vi "FPGA upload data to LEDs.vi"() -> ()   [LabVIEW 2016]
uses:
  Program Files (x86)/National Instruments/LabVIEW 2016/examples/roboRIO/Customized FPGA/Sub VIs/Utilities/Start Boolean.ctl
  <vilib>/Platform/TimedLoop/XDataNode/timing_clust.ctl
  <vilib>/Platform/TimedLoop/XDataNode/nitl_modes.ctl
  <vilib>/Platform/TimedLoop/XDataNode/wakeup.ctl
  <vilib>/rvi/Emulation/niFpgaGetClockAttributes.vi
  <vilib>/rvi/Emulation/niFpgaSctlEmulationGetInTimedLoop.vi
  <vilib>/rvi/Emulation/niFpgaEmulationReportErrorSimple.vi
  <vilib>/rvi/eio/common/nirviEmuTemplateMethod_errors.vi
  <vilib>/rvi/Emulation/niFpgaCriticalErrorInLSC.vi
  <vilib>/rvi/Emulation/niFpgaProcessEmulError.vi
  <vilib>/rvi/Emulation/niFpgaEmulationIsFPGAContextNoSignature.vi
  <vilib>/rvi/errors/niFpgaSetErrorForExecOnDevCompSimple.vi
  <vilib>/rvi/eio/common/nirviEmuReportErrorAndStop.vi
  <vilib>/rvi/DataTransferAndStorage/Container/Common/niFpgaContainerGetUniqueNameForEmu.vi
  <vilib>/rvi/FIFO/Fifo_Resource/nirvififoEmulationSetSize.vi
  <vilib>/rvi/FIFO/Fifo_Resource/nirviFifoEmulationQueueMgr.vi
  <instcachedir>/0/nirviFifoEmulationQueueMgr_E5CAEC123FF24DC58D834DCA3CDAA9B5.lvgen/nirviFifoEmulationQueueMgr_E5CAEC123FF24DC58D834DCA3CDAA9B5_000.vi
  <vilib>/Utility/error.llb/Clear Errors.vi
  <vilib>/rvi/FIFO/Fifo_Resource/nirvififoEmulationCreateLock.vi
  <vilib>/rvi/FIFO/Fifo_Resource/nirvififoEmulationObtainLock.vi
  <vilib>/rvi/FIFO/Fifo_Resource/nirvififoEmulationReleaseLock.vi
  <vilib>/rvi/occurrence/nirviWaitOnOccurrenceBase.vi
  <vilib>/rvi/errors/nirviReportUnexpectedCaseInternalError.vi
  <vilib>/rvi/errors/nirviReportUnexpectedCaseInternalError (U32).vi
  <vilib>/rvi/FIFO/Fifo_Resource/nirvififoEmulationDetermineInputValidOut.vi
  <vilib>/rvi/DataTransferAndStorage/Container/Common/niFpgaContainerSetEmuInfo.vi
  <vilib>/rvi/DataTransferAndStorage/Container/Common/niFpgaContainerExecOnDevCompGetState.vi
  <instcachedir>/0/nirviFifoEmulationQueueMgr_E5CAEC123FF24DC58D834DCA3CDAA9B5.lvgen/nirviFifoEmulationQueueMgr_E5CAEC123FF24DC58D834DCA3CDAA9B5_003.vi
  <vilib>/rvi/interface/RandomDataEmulation/niFpgaRandomDataHandleErrors.vi
  <vilib>/eio/EIONode/EIONode.xnode
  <vilib>/rvi/DataTransferAndStorage/Container/XNode/niFpgaContainer.xnode
  <vilib>/rvi/FIFO/Fifo_Resource/nirvififoEmulationRead.vi
  <vilib>/rvi/FIFO/Fifo_Resource/nirvififoEmulationWrite.vi
  <vilib>/rvi/LocalResourceManager/LocalResourceManager.xnode
  <vilib>/rvi/FIFO/Fifo_Resource/niFpgaFifoEmulationRefIn.vi
  <vilib>/Platform/TimedLoop/XDataNode/XDataNode.xnode
  <vilib>/Platform/TimedLoop/XDataNode/XDNodeRunTimeDep.lvlib
panel:
  in  "SYS.SELECTB":u8 format="%08b"
  in  "DIO.B_7:0.OUT":u8 format="%08b"
  in  "DIO.B_7:0.DIR":u8 format="%08b"
  out "DIO.B_7:0.IN":u8 format="%08b"
  in  "DIO.B_15:8.OUT":u8 format="%08b"
  in  "DIO.B_15:8.DIR":u8 format="%08b"
  out "DIO.B_15:8.IN":u8 format="%08b"
  in  "SPI.B.DATO":u16
  out "SPI.B.DATI":u16
  in  "SPI.B.CNFG":u16 format="%016b"
  in  "SPI.B.CNT":u16
  in  "SPI.B.GO":T1
  out "SPI.B.STAT":u8 format="%08b"
  in  "PWM.B_0.MAX":u16
  in  "PWM.B_0.CMP":u16
  in  "PWM.B_0.CNFG":u8 format="%08b"
  in  "PWM.B_0.CS":u8
  out "PWM.B_0.CNTR":u16
  in  "PWM.B_1.CMP":u16
  in  "PWM.B_1.MAX":u16
  out "PWM.B_1.CNTR":u16
  in  "PWM.B_1.CNFG":u8 format="%08b"
  in  "PWM.B_1.CS":u8
  in  "PWM.B_2.CMP":u16
  in  "PWM.B_2.MAX":u16
  out "PWM.B_2.CNTR":u16
  in  "PWM.B_2.CNFG":u8 format="%08b"
  in  "PWM.B_2.CS":u8
  in  "I2C.B.DATO":u8
  out "I2C.B.DATI":u8
  in  "I2C.B.ADDR":u8 format="%08b"
  in  "I2C.B.CNTR":u8
  in  "I2C.B.CNTL":u8 format="%08b"
  out "I2C.B.STAT":u8 format="%08b"
  in  "I2C.B.CNFG":u8 format="%08b"
  in  "I2C.B.GO":T1
  in  "ENC.B.CNFG":u8 format="%08b"
  out "ENC.B.CNTR":u32
  out "ENC.B.STAT":u8 format="%08b"
  in  "SPI.B.IRQ.NO":u8=15
  in  "IRQ.DIO_B_7:0.ENA":u8 format="%08b"
  in  "IRQ.DIO_B_7:0.RISE":u8 format="%08b"
  in  "IRQ.DIO_B_7:0.FALL":u8 format="%08b"
  in  "IRQ.DIO_B_0.CNT":u32
  in  "IRQ.DIO_B_1.CNT":u32
  in  "IRQ.DIO_B_2.CNT":u32
  in  "IRQ.DIO_B_3.CNT":u32
  in  "IRQ.DIO_B_3.NO":u8
  in  "IRQ.DIO_B_2.NO":u8
  in  "IRQ.DIO_B_1.NO":u8
  in  "IRQ.DIO_B_0.NO":u8
  out "AI.B_0.VAL":u16
  out "AI.B_1.VAL":u16
  out "AI.B_2.VAL":u16
  out "AI.B_3.VAL":u16
  out "AI.AI_0.VAL":u16
  out "AI.AI_1.VAL":u16
  out "AI.AI_2.VAL":u16
  out "AI.AI_3.VAL":u16
  out "SYS.AI.RDY":bool
  in  "IRQ.AI_B_3:0.CNFG":u8 format="%.0b"
  in  "IRQ.AI_B_0.THRESHOLD":u16
  in  "IRQ.AI_B_1.THRESHOLD":u16
  in  "IRQ.AI_B_0.NO":u8
  in  "IRQ.AI_B_1.NO":u8
  in  "IRQ.AI_B_1.HYSTERESIS":u16=17
  in  "IRQ.AI_B_0.HYSTERESIS":u16=17
  in  "AO.B_0.VAL":u16
  in  "AO.B_1.VAL":u16
  in  "AO.SYS.GO":T1
  out "AO.SYS.STAT":bool
  in  "PWM.PWM_0.MAX":u16
  in  "PWM.PWM_0.CMP":u16
  in  "PWM.PWM_0.CNFG":u8 format="%08b"
  in  "PWM.PWM_0.CS":u8
  out "PWM.PWM_0.CNTR":u16
  in  "PWM.PWM_1.MAX":u16
  in  "PWM.PWM_1.CMP":u16
  in  "PWM.PWM_1.CNFG":u8 format="%08b"
  in  "PWM.PWM_1.CS":u8
  out "PWM.PWM_1.CNTR":u16
  in  "PWM.PWM_2.MAX":u16
  in  "PWM.PWM_2.CMP":u16
  in  "PWM.PWM_2.CNFG":u8 format="%08b"
  in  "PWM.PWM_2.CS":u8
  out "PWM.PWM_2.CNTR":u16
  in  "PWM.PWM_3.MAX":u16
  in  "PWM.PWM_3.CMP":u16
  in  "PWM.PWM_3.CNFG":u8 format="%08b"
  in  "PWM.PWM_3.CS":u8
  out "PWM.PWM_3.CNTR":u16
  in  "PWM.PWM_4.MAX":u16
  in  "PWM.PWM_4.CMP":u16
  in  "PWM.PWM_4.CNFG":u8 format="%08b"
  in  "PWM.PWM_4.CS":u8
  out "PWM.PWM_4.CNTR":u16
  in  "PWM.PWM_5.MAX":u16
  in  "PWM.PWM_5.CMP":u16
  in  "PWM.PWM_5.CNFG":u8 format="%08b"
  in  "PWM.PWM_5.CS":u8
  out "PWM.PWM_5.CNTR":u16
  in  "PWM.PWM_6.MAX":u16
  in  "PWM.PWM_6.CMP":u16
  in  "PWM.PWM_6.CNFG":u8 format="%08b"
  in  "PWM.PWM_6.CS":u8
  out "PWM.PWM_6.CNTR":u16
  in  "PWM.PWM_7.MAX":u16
  in  "PWM.PWM_7.CMP":u16
  in  "PWM.PWM_7.CNFG":u8 format="%08b"
  in  "PWM.PWM_7.CS":u8
  out "PWM.PWM_7.CNTR":u16
  in  "PWM.PWM_8.MAX":u16
  in  "PWM.PWM_8.CMP":u16
  in  "PWM.PWM_8.CNFG":u8 format="%08b"
  in  "PWM.PWM_8.CS":u8
  out "PWM.PWM_8.CNTR":u16
  in  "PWM.PWM_9.MAX":u16
  in  "PWM.PWM_9.CMP":u16
  in  "PWM.PWM_9.CNFG":u8 format="%08b"
  in  "PWM.PWM_9.CS":u8
  out "PWM.PWM_9.CNTR":u16
  out "SYS.RDY":bool
  in  "DO.RELAY.OUT":u8 format="%08b"
  out "ACC.Z.VAL":u16
  out "ACC.Y.VAL":u16
  out "ACC.X.VAL":u16
  out "SYS.ACC.RDY":bool
  in  "I2C.I2C.DATO":u8
  in  "I2C.I2CADDR":u8 format="%08b"
  in  "I2C.I2C.CNTR":u8
  in  "I2C.I2C.CNTL":u8 format="%08b"
  in  "I2C.I2C.CNFG":u8 format="%08b"
  in  "I2C.I2C.GO":T1
  out "I2C.I2C.DATI":u8
  out "I2C.I2C.STAT":u8 format="%08b"
  in  "SPI.SPI.DATO":u16
  out "SPI.SPI.DATI":u16
  in  "SPI.SPI.CNFG":u16 format="%016b"
  in  "SPI.SPI.CNT":u16
  in  "SPI.SPI.GO":T1
  out "SPI.SPI.STAT":u8 format="%08b"
  in  "SPI.SPI.IRQ.NO":u8=15
  in  "DIO.SPI_CS3:0.OUT":u8 format="%08b"
  in  "DIO.SPI_CS3:0.DIR":u8 format="%08b"
  out "DIO.SPI_CS3:0.IN":u8 format="%08b"
  in  "DO.RSL.OUT":bool
  in  "DO.LED 5:0":u8 format="%06b"
  out "DI.BTN":u8 format="%08b"
  in  "IRQ.DI_BTN.ENA":bool
  in  "IRQ.DI_BTN.RISE":bool
  in  "IRQ.DI_BTN.FALL":bool
  in  "IRQ.DI_BTN.CNT":u32
  in  "IRQ.DI_BTN.NO":u8
  in  "IRQ.TIMER.SETTIME":T1
  in  "IRQ.TIMER.WRITE":u32
  out "IRQ.TIMER.READ":u32
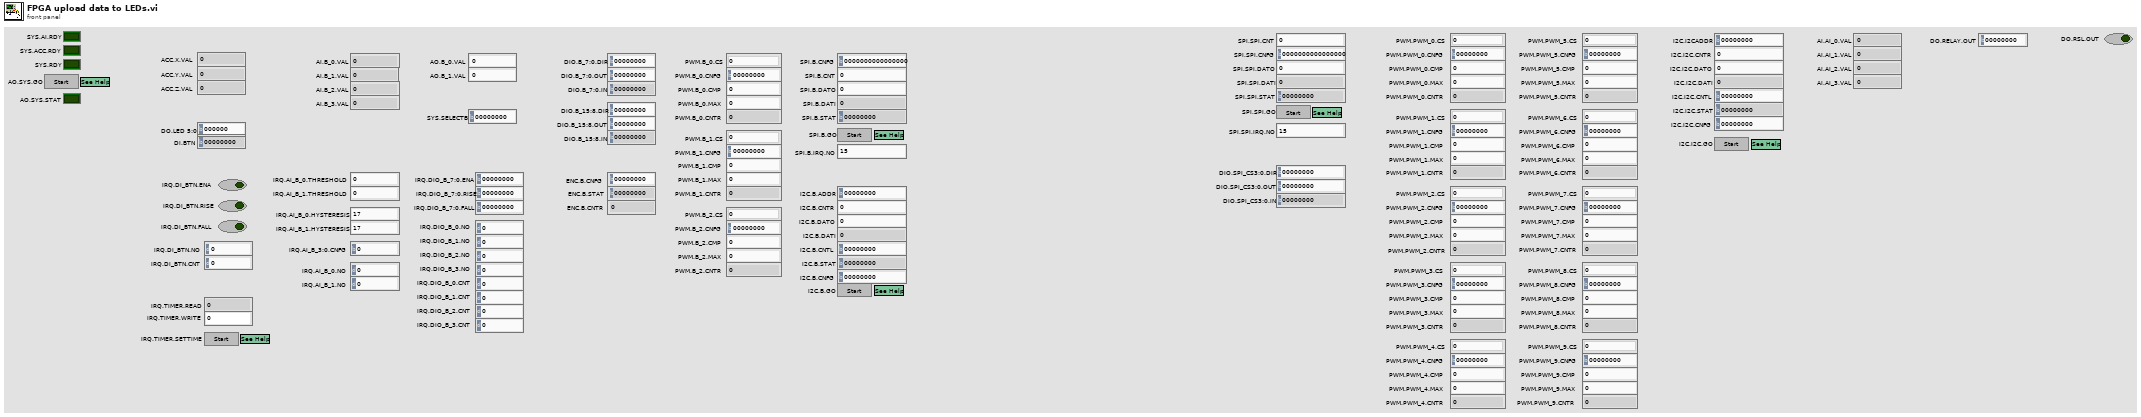
[diagram p1: front panel]
types:
  T1 = typedef "Start Boolean.ctl" = bool
  T2 = typedef "XDNodeRunTimeDep.lvlib/timing_clust.ctl" = cluster{"Expected End [f-1]":u64, "Actual End [f-1]":u64, "Finished Late? [f-1]":bool, "Expected End [i-1]":u64, "Actual End [i-1]":u64, "Finished Late? [i-1]":bool, "Expected Start [i]":u64, "Actual Start [i]":u64, "Expected Start [f]":u64, "Actual Start [f]":u64, "Source Name":string, "Structure Name":string, "Period":i64, "Deadline":i64, "Offset":i64, "Start":i64, "Priority":i32, "Timeout":i32, "Mode":T3, "Wakeup Reason":T4, "Error":errorcluster, "Source Type":string, "Secondary Source Type":string, "Global End Time":u64, "Global Start Time":u64, "Frame Duration":u64, "Iteration Duration":u64, "Assigned CPU":i32, "I/O Scan Engine Mode":u32}
  T3 = typedef "XDNodeRunTimeDep.lvlib/nitl_modes.ctl" = enum32{"No Change", "Process missed periods, maintain original phase", "Discard missed periods, maintain original phase", "Process missed periods, ignore original phase", "Discard missed periods, ignore original phase"}
  T4 = typedef "XDNodeRunTimeDep.lvlib/wakeup.ctl" = enum32{"Normal", "Aborted", "Asynchronous wakeup", "Timing source error", "Timed loop error", "Timeout"}
diagram:
  # "Needed for express VIs and other roboRIO stuff"
  # "Other Code"
  # "LED Code"
  # "The accelerometer nodes take some time before the FPGA can first read the values. This is because it takes time to read from the accelerometer. An iteration of the While Loop will not complete until the accelerometer values have been read.\n\nAfter the completion of the first iteration of the While Loop, all indicators have valid values."
  # "The analog output nodes take some time before the FPGA write the values to the pins. The GO and STAT registers are used to handshake between the FPGA and host. When the host wants the values to be written, the host sets the GO register to TRUE. If the host reads the STAT register before setting the value of the GO register, it can wait for the value of the STAT register to invert. The value inversion tells the host that the output values have been written."
  # "The FPGA timer fires the interrupt request (IRQ) when TIMER.Read counts down to zero. If TIMER.Read is not zero, it counts down to one per microsecond."
  # "The analog input nodes take some time before the FPGA can first read the values. This is because it takes time to set up the Analog-to-Digital converter (ADC) and convert the first reading. An iteration of the While Loop will not complete until all the analog input channels have been sampled.\n\nAfter the completion of the first iteration of the While Loop, all indicators have valid values."
  # "Note: On some hardware a \"ghosting effect\" may occur on any unconnected AI channels. For example, if channel AI0 is connected and channels AI1~AI7 are not connected the the value read at AI0 may be seen on indicators AI1~AI7. This is common for hardware that use a multiplexed (MUXed) Analog-to-Digital converter (ADC), because the input analog signal is used to charge a capacitor which does not discharge before the unconnected channel is read.\n\nYou can hide the \"ghosting effect\" by using an mask register. This register is used to decide when the indicator should be updated."
  # "The only interface that sends interrupts to the RT side. Timer interrupts, analog input interrupts, digital input interrupts, and SPI interrupt share this interface.\n\nAll interrupts work in sequence. One interrupt waits until the previous interrupt request (IRQ) gets acknowledged on the RT side."
  # "NOTE: The SYS.RDY boolean MUST exist and must become TRUE at some point otherwise the myRIO API will not function correctly."
  # "There is some delay between when the FPGA code starts and the analog inputs, accelerometer, and scaling values outputs are valid. If the host wants to ensure that there are valid values in theses registers it should wait for each subsystem to finish its initialization process. \n\nWhen all subsystems have finished initializinig, the SYS.RDY indicator will be true, which can be polled by the host to determine the status of the FPGA. Alternatively, the host can poll the individual SYS.xx.RDY indicators to determine the status of the individual subsystems.\n\nThis loop continues indefinitely, essentially making SYS.RDY a read-only register."
  # "Inbound DMA FIFO from host"
  # "Pushes data out to LED string"
  # "Physical line"
  # "ID"
  # "Inbound data contains a reset bit,\n7 ID code bits and 24 colour bits\nmsb                                            lsb\nRiiiiiiirrrrrrrrggggggggbbbbbbbb"
  n1 = xnode "VI-Defined FIFO Configuration"() -> ("FIFO Out"=w24:refnum<k21>)
  n2 = xnode "VI-Defined FIFO Configuration"() -> ("FIFO Out"=w25:refnum<k21>)
  n3 = xnode "VI-Defined FIFO Configuration"() -> ("FIFO Out"=w26:refnum<k21>)
  n4 = xnode "VI-Defined FIFO Configuration"() -> ("FIFO Out"=w27:refnum<k21>)
  n5 = call "FPGA Control of one WS2812 string.vi"("FPGA DO line"=refnum<k21> "DIO/DIO0" ("FPGA I/O In"), "Wire ID"=u8 1 ("ID"), "FIFO In"=w27) -> ()  [unwired: 9 in]
  n6 = call "FPGA Control of one WS2812 string.vi"("FPGA DO line"=refnum<k21> "DIO/DIO1" ("FPGA I/O In"), "Wire ID"=u8 2 ("ID"), "FIFO In"=w26) -> ()  [unwired: 9 in]
  n7 = call "FPGA Control of one WS2812 string.vi"("FPGA DO line"=refnum<k21> "DIO/DIO2" ("FPGA I/O In"), "Wire ID"=u8 3 ("ID"), "FIFO In"=w25) -> ()  [unwired: 9 in]
  n8 = call "FPGA Control of one WS2812 string.vi"("FPGA DO line"=refnum<k21> "DIO/DIO3" ("FPGA I/O In"), "Wire ID"=u8 4 ("ID"), "FIFO In"=w24) -> ()  [unwired: 9 in]
  n9 = while {
    tunnel: refnum<k21> "LED data to FPGA FIFO" ("FIFO In") -> [w41]
    tunnel: w27 -> [w39]
    tunnel: w26 -> [w38]
    tunnel: w25 -> [w37]
    tunnel: w24 -> [w36]
    shift-right: [w34] -> _
    shift-left: _ -> [w33]
    stop <- FALSE stop-if-true
    w35 = -1 ("Timeout")
    # "Pass inbound data to every drive VI"
    n10 = xnode ("FIFO Write")("Element"=w33, "Timeout"=w35, "FIFO In"=w36) -> ()  [unwired: 2 out]
    n11 = xnode ("FIFO Write")("Element"=w33, "Timeout"=w35, "FIFO In"=w37) -> ()  [unwired: 2 out]
    n12 = xnode ("FIFO Write")("Element"=w33, "Timeout"=w35, "FIFO In"=w38) -> ()  [unwired: 2 out]
    n13 = xnode ("FIFO Write")("Element"=w33, "Timeout"=w35, "FIFO In"=w39) -> ()  [unwired: 2 out]
    n14 = xnode ("FIFO Read")("Timeout"=w35, "FIFO In"=w41) -> ("Element"=w34:u32)  [unwired: 2 out]
  }
  n15 = while {
    stop <- FALSE stop-if-true
    # "Host Synchronization"
    n16 = local read "SYS.ACC.RDY"() -> (w43:bool)
    n17 = local read "SYS.AI.RDY"() -> (w45:bool)
    n18 = Compound Arithmetic op=AND(w45, w43) -> (→"SYS.RDY":bool)
  }
  n19 = while {
    stop <- FALSE stop-if-true
    # "Interrupt to RT"
    n20 = xnode ("FIFO Method Node")("Timeout"=-1) -> ("Element"=w48:u8)  [unwired: 1 in, 2 out]
    n21 = call <vilib>:"niFPGA Interrupt.vi"("Wait Until Cleared (F)"=TRUE, "IRQ Number (0)"=w48) -> ()  [unwired: 1 in]
  }
  n22 = while {
    stop <- FALSE stop-if-true
    # "Timer"
    n23 = local read "IRQ.TIMER.READ"() -> (w53:u32)
    n24 = Select(t="IRQ.TIMER.WRITE", s="IRQ.TIMER.SETTIME", f=w53) -> (s? t:f=w51:u32)
    n25 = case shown="Default" w51 {
      selector: w51 -> [w57 w60]
      tunnel: [w57 w58] -> w50
      frame 0 {
      }
      frame Default {
        n26 = Decrement(x=w60) -> (x-1=w59:u32)
        n27 = case shown="0" w59 {
          selector: w59 -> [w61 w64]
          tunnel: [w61 w64] -> w58
          frame Default {
          }
          frame 0 {
            w63 = u8 0  # Reserved for Timer IRQ
            n28 = xnode ("FIFO Method Node")("Element"=w63, "Timeout"=-1) -> ()  [unwired: 1 in, 2 out]
          }
        }
      }
    }
    "IRQ.TIMER.READ" <- w50
    n29 = call "Loop Timer"("Count(uSec)"=u8 1 ("Count(mSec)")) -> ()  [unwired: 1 out]
  }
  n30 = xnode "VI-Defined FIFO Configuration"() -> ("FIFO Out"=w4:refnum<k21>)
  n31 = while {
    tunnel: w4 -> [w73]
    i -> [w87]
    stop <- FALSE stop-if-true
    # "Analog Input"
    n32 = Greater Than 0?(x=w87) -> (x > 0?=→"SYS.AI.RDY":bool)
    n33 = xnode "FPGA I/O Node"() -> ("MXP/AI0"=w66:u16, "MXP/AI1"=w65:u16, "MXP/AI2"=→"AI.B_2.VAL":u16, "MXP/AI3"=→"AI.B_3.VAL":u16, "AnalogIn0"=→"AI.AI_0.VAL":u16, "AnalogIn1"=→"AI.AI_1.VAL":u16, "AnalogIn2"=→"AI.AI_2.VAL":u16, "AnalogIn3"=→"AI.AI_3.VAL":u16)  [unwired: 8 in, 8 out]
    "AI.B_0.VAL" <- w66
    "AI.B_1.VAL" <- w65
    n34 = Number To Boolean Array(number="IRQ.AI_B_3:0.CNFG") -> (Boolean array=w74:bool[])
    n35 = Index Array(array=w74) -> (element #1=w76:bool, element #2=w77:bool, element #3=w79:bool, element #4=w80:bool)  [unwired: 4 in]
    n36 = call "Check AI IRQ.vi"("Hysteresis"="IRQ.AI_B_1.HYSTERESIS", "FIFO In"=w73, "IRQ Number"="IRQ.AI_B_1.NO", "Threshold"="IRQ.AI_B_1.THRESHOLD", "Analog Value"=w65, "Rising Edge?"=w80, "Enable Interrupt?"=w79) -> ()  [unwired: 5 in]
    n37 = call "Check AI IRQ.vi"("Hysteresis"="IRQ.AI_B_0.HYSTERESIS", "FIFO In"=w73, "IRQ Number"="IRQ.AI_B_0.NO", "Threshold"="IRQ.AI_B_0.THRESHOLD", "Analog Value"=w66, "Rising Edge?"=w77, "Enable Interrupt?"=w76) -> ()  [unwired: 5 in]
  }
  n38 = while {
    stop <- FALSE stop-if-true
    # "Analog Output"
    n39 = feedback #1(FALSE) -> (w91:bool)
    n40 = case shown="True" "AO.SYS.GO" {
      tunnel: "AO.B_0.VAL" -> [_ w101]
      tunnel: "AO.B_1.VAL" -> [_ w100]
      tunnel: w91 -> [w96 w99]
      tunnel: [w96 w97] -> w89
      frame False {
      }
      frame True {
        n41 = flat-sequence {
          tunnel: w101 -> [w104]
          tunnel: w100 -> [w103]
          tunnel: w99 -> [w102]
          tunnel: [w102] -> w98
          tunnel: w98 -> [w106]
          tunnel: [w105] -> w97
          frame #0 {
            n42 = xnode "FPGA I/O Node"("MXP/AO0"=w104, "MXP/AO1"=w103) -> ()  [unwired: 2 in, 2 out]
          }
          frame #1 {
            n43 = Not(x=w106) -> (.not. x?=w105:bool)
          }
        }
      }
    }
    "AO.SYS.STAT" <- w89
    n44 = feedback-in #1(w89) -> ()
  }
  n45 = while {
    i -> [w114]
    stop <- FALSE stop-if-true
    # "Onboard Accelerometer"
    n46 = xnode "FPGA I/O Node"() -> ("AccelerationX"=w112:i16, "AccelerationY"=w111:i16, "AccelerationZ"=w110:i16)  [unwired: 3 in, 3 out]
    n47 = Greater Than 0?(x=w114) -> (x > 0?=→"SYS.ACC.RDY":bool)
    n48 = To Unsigned Word Integer(number=w112) -> (unsigned 16bit integer=→"ACC.X.VAL":u16)
    n49 = To Unsigned Word Integer(number=w111) -> (unsigned 16bit integer=→"ACC.Y.VAL":u16)
    n50 = To Unsigned Word Integer(number=w110) -> (unsigned 16bit integer=→"ACC.Z.VAL":u16)
  }
  n51 = xnode "VI-Defined FIFO Configuration"() -> ("FIFO Out"=w5:refnum<k21>)
  n52 = node-c288() -> (w7:T2)  [unwired: 1 in]
  n53 = timed-loop {
    timing: w7 -> [_]
    timing-out: [_] -> w6
    tunnel: w5 -> [w121]
    stop <- FALSE stop-if-true
    # "Button IRQ"
    # "Onboard DIO"
    n54 = xnode "FPGA I/O Node"() -> ("User Button"=w122:bool)  [unwired: 1 in, 1 out]
    n55 = Number To Boolean Array(number="DO.LED 5:0") -> (Boolean array=w132:bool[])
    n56 = Index Array(array=w132) -> (element #1=w130:bool, element #2=w129:bool, element #3=w128:bool, element #4=w127:bool, element #5=w126:bool, element #6=w125:bool)  [unwired: 6 in]
    n57 = Build Array(w122) -> (w124:bool[])
    n58 = call "DIO IRQ 1-bit.vi"("IRQ.NO"="IRQ.DI_BTN.NO", "IRQ.CNT"="IRQ.DI_BTN.CNT", "FIFO in"=w121, "IRQ.FALL"="IRQ.DI_BTN.FALL", "IRQ.RISE"="IRQ.DI_BTN.RISE", "IRQ.ENA"="IRQ.DI_BTN.ENA", "DIO"=w122) -> ()  [unwired: 5 in]
    n59 = Boolean Array To Number(Boolean array=w124) -> (number=→"DI.BTN":u8)
    n60 = xnode "FPGA I/O Node"("Radio LED Green"=w130, "Radio LED Red"=w129, "Comm LED Green"=w128, "Comm LED Red"=w127, "Mode LED Green"=w126, "Mode LED Red"=w125) -> ()  [unwired: 6 in, 6 out]
  }
  n61 = while {
    stop <- FALSE stop-if-true
    # "Button SCTL Interrupt Buffer"
    n62 = feedback #2(u8 0 ("Element")) -> (w138:u8)
    n63 = feedback #3(FALSE ("Timed Out?")) -> (w142:bool)
    n64 = case shown="False" w142 {
      tunnel: [w144 w146] -> w139
      tunnel: w138 -> [_ w146]
      frame False {
        n65 = xnode ("FIFO Read")("Timeout"=-1) -> ("Element"=w144:u8)  [unwired: 1 in, 2 out]
      }
      frame True {
      }
    }
    n66 = feedback-in #2(w139) -> ()
    n67 = xnode ("FIFO Method Node")("Element"=w139, "Timeout"=0) -> ("Timed Out?"=w140:bool)  [unwired: 1 in, 1 out]
    n68 = feedback-in #3(w140) -> ()
  }
  n69 = node-c288(w6) -> ()
  n70 = xnode "VI-Defined FIFO Configuration"() -> ("FIFO Out"=w1:refnum<k21>)
  n71 = xnode "VI-Defined FIFO Configuration"() -> ("FIFO Out"=w3:refnum<k21>)
  n72 = node-c288() -> (w19:T2)  [unwired: 1 in]
  n73 = timed-loop {
    timing: w19 -> [_]
    timing-out: [_] -> w18
    tunnel: w1 -> [w183]
    tunnel: w3 -> [w171]
    stop <- _ stop-if-true
    # "DIO/ IRQ"
    # "DIO / Encoder"
    # "DIO / I2C Master"
    # "DIO / PWM"
    # "DIO"
    # "DIO"
    # "DIO/ SPI Master"
    # "Connector MXP DIO"
    n74 = call "Split HDC Bank1 DIO.vi"("IN 7:0"="DIO.B_7:0.OUT") -> ("OUT 3:0"=w271:fxp<+,4,4>, "OUT 4"=w186:bool, "OUT 7:5"=w268:fxp<+,3,3>)
    n75 = call "Split HDC Bank1 DIO.vi"("IN 7:0"="DIO.B_7:0.DIR") -> ("OUT 3:0"=w270:fxp<+,4,4>, "OUT 4"=w269:bool, "OUT 7:5"=w267:fxp<+,3,3>)
    n76 = call "Split HDC Function Select.vi"("IN 7:0"="SYS.SELECTB") -> ("OUT 1:0"=w207:fxp<+,2,2>, "OUT 7"=w202:bool, "OUT 2"=w206:bool, "OUT 3"=w205:bool, "OUT 4"=w204:bool, "OUT 5"=w203:bool)
    n77 = call "DIO 4-bit.vi"("DIO0 Refnum"=refnum<k21> "MXP/DIO0", "DIO1 Refnum"=refnum<k21> "MXP/DIO1", "DIO2 Refnum"=refnum<k21> "MXP/DIO2", "DIR 3:0"=w270, "OUT 3:0"=w271, "DIO3 Refnum"=refnum<k21> "MXP/DIO3") -> ("IN 3:0"=w182:fxp<+,4,4>)  [unwired: 5 in]
    n78 = call "DIO 1-bit.vi"("DIR"=w269, "OUT"=w186, "DIO Refnum"=refnum<k21> "MXP/DIO4") -> ("IN"=w243:bool)  [unwired: 8 in]
    n79 = call "DIO_SPI.vi"("DIO.2:0.OUT"=w268, "DIO.2:0.DIR"=w267, "SPI.CNT"="SPI.B.CNT", "SPI.CNFG"="SPI.B.CNFG", "SPI.DATO"="SPI.B.DATO", "SPI.GO"="SPI.B.GO", "DIO.2/SPI.MOSI Refnum"=refnum<k21> "MXP/DIO7" ("DIO.2/SPI.SCLK"), "SELECT.1:0"=w207, "DIO.1/SPI.MISO Refnum"=refnum<k21> "MXP/DIO6" ("DIO.1/SPI.MOSI"), "DIO.0/SPI.SCLK Refnum"=refnum<k21> "MXP/DIO5" ("DIO.0/SPI.MISO")) -> ("DIO.2:0.IN"=w242:fxp<+,3,3>, "SPI.DATI"=→"SPI.B.DATI":u16, "SPI.STAT"=w185:u8)  [unwired: 7 in]
    "SPI.B.STAT" <- w185
    n80 = call "SPI IRQ.vi"("SPI.A.IRQ.NO"="SPI.B.IRQ.NO", "SPI.STAT"=w185, "FIFO In"=w183) -> ()  [unwired: 9 in]
    n81 = call "Join HDC Bank1 DIO.vi"("IN 7:5"=w242, "IN 4"=w243, "IN 3:0"=w182) -> ("OUT 7:0"=→"DIO.B_7:0.IN":u8)
    n82 = Number To Boolean Array(number="IRQ.DIO_B_7:0.ENA") -> (Boolean array=w168:bool[])
    n83 = Number To Boolean Array(number="IRQ.DIO_B_7:0.RISE") -> (Boolean array=w159:bool[])
    n84 = Number To Boolean Array(number="IRQ.DIO_B_7:0.FALL") -> (Boolean array=w154:bool[])
    n85 = Index Array(array=w168) -> (element #1=w169:bool, element #2=w167:bool, element #3=w166:bool, element #4=w165:bool)  [unwired: 4 in]
    n86 = Index Array(array=w159) -> (element #1=w158:bool, element #2=w160:bool, element #3=w161:bool, element #4=w162:bool)  [unwired: 4 in]
    n87 = Index Array(array=w154) -> (element #1=w155:bool, element #2=w153:bool, element #3=w152:bool, element #4=w151:bool)  [unwired: 4 in]
    n88 = Build Array(w169, w167, w166, w165) -> (w170:bool[])
    n89 = Build Array(w158, w160, w161, w162) -> (w157:bool[])
    n90 = Build Array(w155, w153, w152, w151) -> (w156:bool[])
    n91 = Build Array("IRQ.DIO_B_0.CNT", "IRQ.DIO_B_1.CNT", "IRQ.DIO_B_2.CNT", "IRQ.DIO_B_3.CNT") -> (w177:u32[])
    n92 = Build Array("IRQ.DIO_B_0.NO", "IRQ.DIO_B_1.NO", "IRQ.DIO_B_2.NO", "IRQ.DIO_B_3.NO") -> (w172:u8[])
    n93 = Boolean Array To Number(Boolean array=w170) -> (number=w163:fxp<+,4,4>)
    n94 = Boolean Array To Number(Boolean array=w157) -> (number=w148:fxp<+,4,4>)
    n95 = Boolean Array To Number(Boolean array=w156) -> (number=w147:fxp<+,4,4>)
    n96 = call "DIO IRQ 4-bit.vi"("IRQ NO"=w172, "IRQ CNT"=w177, "FIFO In"=w171, "IRQ.FALL"=w147, "IRQ.RISE"=w148, "IRQ.ENA"=w163, "IN 3:0"=w182) -> ()  [unwired: 5 in]
    n97 = call "Split HDC Bank2 DIO.vi"("IN 7:0"="DIO.B_15:8.OUT") -> ("OUT 5"=w188:bool, "OUT 7:6"=w212:fxp<+,2,2>, "OUT 4:3"=w190:fxp<+,2,2>, "OUT 2"=w192:bool, "OUT 0"=w196:bool, "OUT 1"=w195:bool)  [unwired: 2 in]
    n98 = call "Split HDC Bank2 DIO.vi"("IN 7:0"="DIO.B_15:8.DIR") -> ("OUT 5"=w187:bool, "OUT 7:6"=w211:fxp<+,2,2>, "OUT 4:3"=w189:fxp<+,2,2>, "OUT 2"=w191:bool, "OUT 0"=w194:bool, "OUT 1"=w193:bool)  [unwired: 2 in]
    n99 = call "DIO_PWM.vi"("DIO.OUT"=w196, "DIO.DIR"=w194, "PWM.CS"="PWM.B_0.CS", "PWM.CNFG"="PWM.B_0.CNFG", "PWM.CMP"="PWM.B_0.CMP", "PWM.MAX"="PWM.B_0.MAX", "DIO/PWM"=refnum<k21> "MXP/DIO8", "SELECT"=w206) -> ("DIO.IN"=w201:bool, "PWM.CNTR"=→"PWM.B_0.CNTR":u16)  [unwired: 10 in]
    n100 = call "DIO_PWM.vi"("DIO.OUT"=w195, "DIO.DIR"=w193, "PWM.CS"="PWM.B_1.CS", "PWM.CNFG"="PWM.B_1.CNFG", "PWM.CMP"="PWM.B_1.CMP", "PWM.MAX"="PWM.B_1.MAX", "DIO/PWM"=refnum<k21> "MXP/DIO9", "SELECT"=w205) -> ("DIO.IN"=w200:bool, "PWM.CNTR"=→"PWM.B_1.CNTR":u16)  [unwired: 10 in]
    n101 = call "DIO_PWM.vi"("DIO.OUT"=w192, "DIO.DIR"=w191, "PWM.CS"="PWM.B_2.CS", "PWM.CNFG"="PWM.B_2.CNFG", "PWM.CMP"="PWM.B_2.CMP", "PWM.MAX"="PWM.B_2.MAX", "DIO/PWM"=refnum<k21> "MXP/DIO10", "SELECT"=w204) -> ("DIO.IN"=w199:bool, "PWM.CNTR"=→"PWM.B_2.CNTR":u16)  [unwired: 10 in]
    n102 = call "DIO_Encoder.vi"("DIO.1:0.OUT"=w190, "DIO.1:0.DIR"=w189, "QE.CNFG"="ENC.B.CNFG", "DIO.1/QE.B"=refnum<k21> "MXP/DIO12", "SELECT"=w203, "DIO.0/QE.A"=refnum<k21> "MXP/DIO11") -> ("DIO.1:0.IN"=w198:fxp<+,2,2>, "QE.CNTR"=→"ENC.B.CNTR":u32, "QE.STAT"=→"ENC.B.STAT":u8)  [unwired: 11 in]
    n103 = call "DIO 1-bit.vi"("DIR"=w187, "OUT"=w188, "DIO Refnum"=refnum<k21> "MXP/DIO13") -> ("IN"=w197:bool)  [unwired: 8 in]
    n104 = call "DIO_I2C.vi"("DIO.1:0.OUT"=w212, "DIO.1:0.DIR"=w211, "I2C.CNFG"="I2C.B.CNFG", "I2C.CNTL"="I2C.B.CNTL", "I2C.ADDR"="I2C.B.ADDR", "I2C.DATO"="I2C.B.DATO", "DIO.1/I2C.SDA"=refnum<k21> "MXP/DIO15" ("DIO.1/I2C.SCL"), "I2C.CNTR"="I2C.B.CNTR", "DIO.0/I2C.SCL"=refnum<k21> "MXP/DIO14" ("DIO.0/I2C.SDA"), "Execute?"="I2C.B.GO", "SELECT"=w202) -> ("DIO.1:0.IN"=w209:fxp<+,2,2>, "I2C.DATI"=→"I2C.B.DATI":u8, "I2C.STAT"=→"I2C.B.STAT":u8)  [unwired: 6 in]
    n105 = call "Join HDC Bank2 DIO.vi"("IN 7:6"=w209, "IN 5"=w197, "IN 4:3"=w198, "IN 0"=w201, "IN 2"=w199, "IN 1"=w200) -> ("OUT 7:0"=→"DIO.B_15:8.IN":u8)  [unwired: 4 in]
  }
  n106 = while {
    stop <- FALSE stop-if-true
    # "Connector A SPI SCTL Interrupt Buffer"
    n107 = feedback #4(u8 0 ("Element")) -> (w276:u8)
    n108 = feedback #5(FALSE ("Timed Out?")) -> (w280:bool)
    n109 = case shown="False" w280 {
      tunnel: [w282 w284] -> w277
      tunnel: w276 -> [_ w284]
      frame False {
        n110 = xnode ("FIFO Method Node")("Timeout"=-1) -> ("Element"=w282:u8)  [unwired: 1 in, 2 out]
      }
      frame True {
      }
    }
    n111 = feedback-in #4(w277) -> ()
    n112 = xnode ("FIFO Method Node")("Element"=w277, "Timeout"=0) -> ("Timed Out?"=w278:bool)  [unwired: 1 in, 1 out]
    n113 = feedback-in #5(w278) -> ()
  }
  n114 = while {
    stop <- FALSE stop-if-true
    # "Connector A DIO SCTL Interrupt Buffer"
    n115 = feedback #6(u8 0 ("Element")) -> (w287:u8)
    n116 = feedback #7(FALSE ("Timed Out?")) -> (w291:bool)
    n117 = case shown="False" w291 {
      tunnel: [w293 w295] -> w288
      tunnel: w287 -> [_ w295]
      frame False {
        n118 = xnode ("FIFO Method Node")("Timeout"=-1) -> ("Element"=w293:u8)  [unwired: 1 in, 2 out]
      }
      frame True {
      }
    }
    n119 = feedback-in #6(w288) -> ()
    n120 = xnode ("FIFO Method Node")("Element"=w288, "Timeout"=0) -> ("Timed Out?"=w289:bool)  [unwired: 1 in, 1 out]
    n121 = feedback-in #7(w289) -> ()
  }
  n122 = node-c288(w18) -> ()
  n123 = node-c288() -> (w17:T2)  [unwired: 1 in]
  n124 = timed-loop {
    timing: w17 -> [_]
    timing-out: [_] -> w16
    stop <- FALSE stop-if-true
    # "PWM"
    n125 = call "PWM (Single Output).vi"("Clock Select"="PWM.PWM_0.CS", "Counter Control"="PWM.PWM_0.CNFG", "Output Compare Value"="PWM.PWM_0.CMP", "Max Counter Value"="PWM.PWM_0.MAX") -> ("Output"=w351:bool, "Counter Value"=→"PWM.PWM_0.CNTR":u16)  [unwired: 6 in]
    n126 = call "PWM (Single Output).vi"("Clock Select"="PWM.PWM_1.CS", "Counter Control"="PWM.PWM_1.CNFG", "Output Compare Value"="PWM.PWM_1.CMP", "Max Counter Value"="PWM.PWM_1.MAX") -> ("Output"=w345:bool, "Counter Value"=→"PWM.PWM_1.CNTR":u16)  [unwired: 6 in]
    n127 = call "PWM (Single Output).vi"("Clock Select"="PWM.PWM_2.CS", "Counter Control"="PWM.PWM_2.CNFG", "Output Compare Value"="PWM.PWM_2.CMP", "Max Counter Value"="PWM.PWM_2.MAX") -> ("Output"=w329:bool, "Counter Value"=→"PWM.PWM_2.CNTR":u16)  [unwired: 6 in]
    n128 = call "PWM (Single Output).vi"("Clock Select"="PWM.PWM_3.CS", "Counter Control"="PWM.PWM_3.CNFG", "Output Compare Value"="PWM.PWM_3.CMP", "Max Counter Value"="PWM.PWM_3.MAX") -> ("Output"=w328:bool, "Counter Value"=→"PWM.PWM_3.CNTR":u16)  [unwired: 6 in]
    n129 = call "PWM (Single Output).vi"("Clock Select"="PWM.PWM_4.CS", "Counter Control"="PWM.PWM_4.CNFG", "Output Compare Value"="PWM.PWM_4.CMP", "Max Counter Value"="PWM.PWM_4.MAX") -> ("Output"=w327:bool, "Counter Value"=→"PWM.PWM_4.CNTR":u16)  [unwired: 6 in]
    n130 = xnode "FPGA I/O Node"("PWM/PWM0"=w351, "PWM/PWM1"=w345, "PWM/PWM2"=w329, "PWM/PWM3"=w328, "PWM/PWM4"=w327) -> ()  [unwired: 5 in, 5 out]
    n131 = call "PWM (Single Output).vi"("Clock Select"="PWM.PWM_5.CS", "Counter Control"="PWM.PWM_5.CNFG", "Output Compare Value"="PWM.PWM_5.CMP", "Max Counter Value"="PWM.PWM_5.MAX") -> ("Output"=w302:bool, "Counter Value"=→"PWM.PWM_5.CNTR":u16)  [unwired: 6 in]
    n132 = call "PWM (Single Output).vi"("Clock Select"="PWM.PWM_6.CS", "Counter Control"="PWM.PWM_6.CNFG", "Output Compare Value"="PWM.PWM_6.CMP", "Max Counter Value"="PWM.PWM_6.MAX") -> ("Output"=w308:bool, "Counter Value"=→"PWM.PWM_6.CNTR":u16)  [unwired: 6 in]
    n133 = call "PWM (Single Output).vi"("Clock Select"="PWM.PWM_7.CS", "Counter Control"="PWM.PWM_7.CNFG", "Output Compare Value"="PWM.PWM_7.CMP", "Max Counter Value"="PWM.PWM_7.MAX") -> ("Output"=w324:bool, "Counter Value"=→"PWM.PWM_7.CNTR":u16)  [unwired: 6 in]
    n134 = call "PWM (Single Output).vi"("Clock Select"="PWM.PWM_8.CS", "Counter Control"="PWM.PWM_8.CNFG", "Output Compare Value"="PWM.PWM_8.CMP", "Max Counter Value"="PWM.PWM_8.MAX") -> ("Output"=w325:bool, "Counter Value"=→"PWM.PWM_8.CNTR":u16)  [unwired: 6 in]
    n135 = call "PWM (Single Output).vi"("Clock Select"="PWM.PWM_9.CS", "Counter Control"="PWM.PWM_9.CNFG", "Output Compare Value"="PWM.PWM_9.CMP", "Max Counter Value"="PWM.PWM_9.MAX") -> ("Output"=w326:bool, "Counter Value"=→"PWM.PWM_9.CNTR":u16)  [unwired: 6 in]
    n136 = xnode "FPGA I/O Node"("PWM/PWM5"=w302, "PWM/PWM6"=w308, "PWM/PWM7"=w324, "PWM/PWM8"=w325, "PWM/PWM9"=w326) -> ()  [unwired: 5 in, 5 out]
  }
  n137 = node-c288(w16) -> ()
  n138 = xnode "VI-Defined FIFO Configuration"() -> ("FIFO Out"=w2:refnum<k21>)
  n139 = node-c288() -> (w11:T2)  [unwired: 1 in]
  n140 = timed-loop {
    timing: w11 -> [_]
    timing-out: [_] -> w10
    tunnel: w2 -> [w361]
    stop <- FALSE stop-if-true
    # "SPI / CS DIO"
    # "SPI / SPI"
    # "SPI"
    n141 = xnode "FPGA I/O Node"() -> ("SPI MISO"=w378:bool)  [unwired: 1 in, 1 out]
    n142 = call "SPI Master.vi"("Count"="SPI.SPI.CNT", "Configuration"="SPI.SPI.CNFG", "Start?"="SPI.SPI.GO", "MISO"=w378, "Data Out"="SPI.SPI.DATO") -> ("Status"=w359:u8, "SCLK"=w372:bool, "MOSI"=w373:bool, "Data In"=→"SPI.SPI.DATI":u16)  [unwired: 3 in]
    "SPI.SPI.STAT" <- w359
    n143 = xnode "FPGA I/O Node"("SPI MOSI"=w373, "SPI CLK"=w372) -> ()  [unwired: 2 in, 2 out]
    n144 = call "SPI IRQ.vi"("SPI.A.IRQ.NO"="SPI.SPI.IRQ.NO", "SPI.STAT"=w359, "FIFO In"=w361) -> ()  [unwired: 9 in]
    n145 = call "Split HDC Bank1 DIO.vi"("IN 7:0"="DIO.SPI_CS3:0.OUT") -> ("OUT 3:0"=w368:fxp<+,4,4>)  [unwired: 2 out]
    n146 = call "Split HDC Bank1 DIO.vi"("IN 7:0"="DIO.SPI_CS3:0.DIR") -> ("OUT 3:0"=w367:fxp<+,4,4>)  [unwired: 2 out]
    n147 = call "DIO 4-bit.vi"("DIO0 Refnum"=refnum<k21> "SPI CS0", "DIO1 Refnum"=refnum<k21> "SPI CS1" ("DIO0 Refnum"), "DIO2 Refnum"=refnum<k21> "SPI CS2" ("DIO0 Refnum"), "DIR 3:0"=w367, "OUT 3:0"=w368, "DIO3 Refnum"=refnum<k21> "SPI CS3" ("DIO0 Refnum")) -> ("IN 3:0"=w366:fxp<+,4,4>)  [unwired: 5 in]
    n148 = call "Join HDC Bank1 DIO.vi"("IN 3:0"=w366) -> ("OUT 7:0"=→"DIO.SPI_CS3:0.IN":u8)  [unwired: 2 in]
  }
  n149 = while {
    stop <- FALSE stop-if-true
    # "Connector SPI SPI SCTL Interrupt Buffer"
    n150 = feedback #8(u8 0 ("Element")) -> (w385:u8)
    n151 = feedback #9(FALSE ("Timed Out?")) -> (w389:bool)
    n152 = case shown="False" w389 {
      tunnel: [w391 w393] -> w386
      tunnel: w385 -> [_ w393]
      frame False {
        n153 = xnode ("FIFO Method Node")("Timeout"=-1) -> ("Element"=w391:u8)  [unwired: 1 in, 2 out]
      }
      frame True {
      }
    }
    n154 = feedback-in #8(w386) -> ()
    n155 = xnode ("FIFO Method Node")("Element"=w386, "Timeout"=0) -> ("Timed Out?"=w387:bool)  [unwired: 1 in, 1 out]
    n156 = feedback-in #9(w387) -> ()
  }
  n157 = node-c288(w10) -> ()
  n158 = node-c288() -> (w13:T2)  [unwired: 1 in]
  n159 = timed-loop {
    timing: w13 -> [_]
    timing-out: [_] -> w12
    stop <- FALSE stop-if-true
    # "I2C"
    n160 = call "DIO_I2C.vi"("I2C.CNFG"="I2C.I2C.CNFG", "I2C.CNTL"="I2C.I2C.CNTL", "I2C.ADDR"="I2C.I2CADDR", "I2C.DATO"="I2C.I2C.DATO", "DIO.1/I2C.SDA"=refnum<k21> "I2C SDA" ("FPGA I/O In"), "I2C.CNTR"="I2C.I2C.CNTR", "DIO.0/I2C.SCL"=refnum<k21> "I2C SCL" ("FPGA I/O In"), "Execute?"="I2C.I2C.GO", "SELECT"=TRUE) -> ("I2C.DATI"=→"I2C.I2C.DATI":u8, "I2C.STAT"=→"I2C.I2C.STAT":u8)  [unwired: 8 in, 1 out]
  }
  n161 = node-c288(w12) -> ()
  n162 = node-c288() -> (w15:T2)  [unwired: 1 in]
  n163 = timed-loop {
    timing: w15 -> [_]
    timing-out: [_] -> w14
    stop <- FALSE stop-if-true
    # "Relay"
    n164 = Number To Boolean Array(number="DO.RELAY.OUT") -> (Boolean array=w416:bool[])
    n165 = Index Array(array=w416) -> (element #1=w415:bool, element #2=w414:bool, element #3=w413:bool, element #4=w412:bool, element #5=w411:bool, element #6=w410:bool, element #7=w409:bool, element #8=w408:bool)  [unwired: 8 in]
    n166 = xnode "FPGA I/O Node"("RelayFwd0"=w415, "RelayRev0"=w414, "RelayFwd1"=w413, "RelayRev1"=w412, "RelayFwd2"=w411, "RelayRev2"=w410, "RelayFwd3"=w409, "RelayRev3"=w408) -> ()  [unwired: 8 in, 8 out]
  }
  n167 = node-c288(w14) -> ()
  n168 = node-c288() -> (w9:T2)  [unwired: 1 in]
  n169 = timed-loop {
    timing: w9 -> [_]
    timing-out: [_] -> w8
    stop <- FALSE stop-if-true
    # "RSL"
    n170 = xnode "FPGA I/O Node"("RSL"="DO.RSL.OUT") -> ()  [unwired: 1 in, 1 out]
  }
  n171 = node-c288(w8) -> ()
